vi "ubinary_load_control.vi"(8 "error in":errorcluster, 10 "file (use dialog)":path, 11 "VI":refnum<vi>) -> (0 "error out":errorcluster)   [LabVIEW 2012]
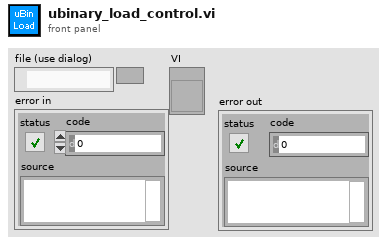
[diagram p1: front panel]
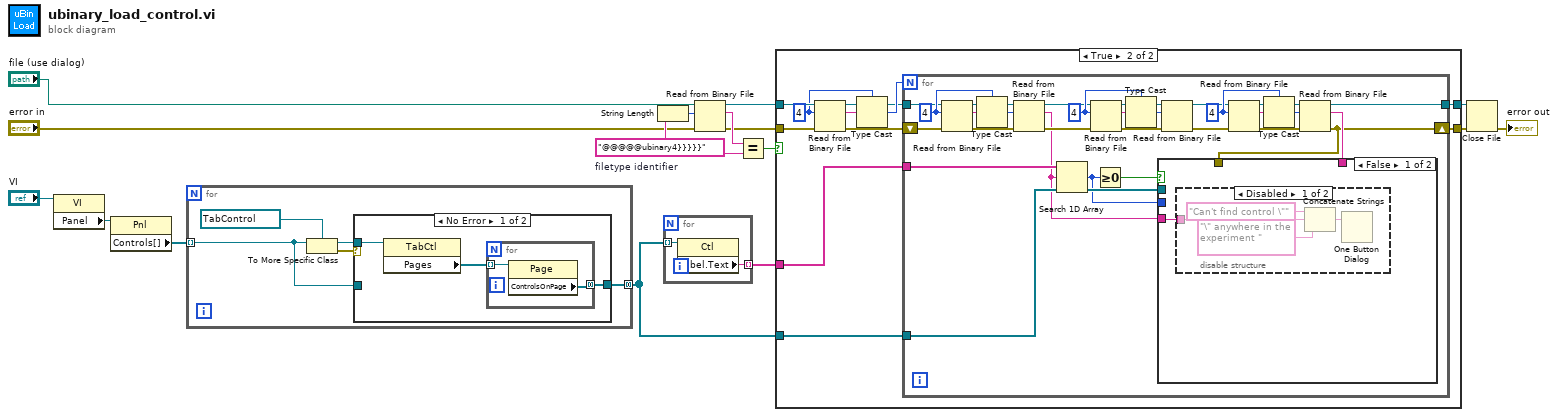
[diagram p0: block diagram]
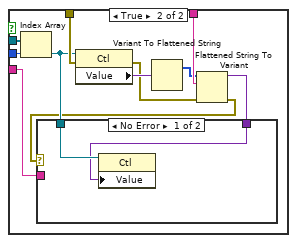
[diagram p4: hidden frame]
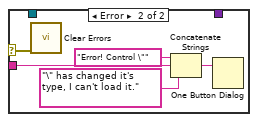
[diagram p5: hidden frame]
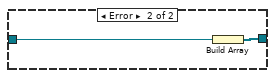
[diagram p6: hidden frame]
diagram:
  w11 = "@@@@@ubinary4}}}}}"  # filetype identifier
  n1 = property class="VI"(reference="VI") -> ("Panel"=w16:refnum<vi>)  [unwired: 1 in, 2 out]
  n2 = property class="Pnl"(reference=w16) -> ("Controls[]"=w15:refnum<vi>[])  [unwired: 1 in, 2 out]
  n3 = for {
    tunnel: w15 -> [w18] mode=indexing
    tunnel: [w17] -> w1 mode=concatenating
    n4 = To More Specific Class(target class=refnum<vi> refnum ("reference"), reference=w18) -> (specific class reference=w20:refnum<vi>, error out=w19:errorcluster)  [unwired: 1 in]
    n5 = case shown="No Error" w19 {
      tunnel: w20 -> [w24 _]
      tunnel: [w22 w28] -> w17
      tunnel: w18 -> [_ w27]
      frame No Error {
        n6 = property on="Property Node" class="TabCtl"(reference=w24) -> ("Pages"=w23:refnum<vi>[])  [unwired: 1 in, 2 out]
        n7 = for {
          tunnel: w23 -> [w26] mode=indexing
          tunnel: [w25] -> w22 mode=concatenating
          n8 = property class="Page"(reference=w26) -> ("ControlsOnPage"=w25:refnum<vi>[])  [unwired: 1 in, 2 out]
        }
      }
      frame Error {
        n9 = Build Array(w27) -> (w28:refnum<vi>[])
      }
    }
  }
  n10 = String Length(string=w11) -> (length=w12:i32)
  n11 = for {
    tunnel: w1 -> [w30] mode=indexing
    tunnel: [w29] -> w6 mode=indexing
    n12 = property class="Ctl"(reference=w30) -> ("Label.Text"=w29:string)  [unwired: 1 in, 2 out]
  }
  n13 = Read from Binary File(8:"error in", 10:w12, 11:"file (use dialog)") -> (0:w7:errorcluster, 2:w10:string, 3:w9:refnum<file>)  [unwired: 3 in, 1 out]
  n14 = Equal?(x=w10, y=w11) -> (x = y?=w8:bool)
  n15 = case shown="True" w8 {
    tunnel: [w32 w33] -> w13
    tunnel: w9 -> [w32 w43]
    tunnel: w7 -> [w31 w38]
    tunnel: w6 -> [_ w37]
    tunnel: [w31 w36] -> w5
    tunnel: w1 -> [_ w35]
    frame False {
    }
    frame True {
      w41 = 4 ("count (1)")
      n16 = Read from Binary File(8:w38, 10:w41, 11:w43) -> (0:w39:errorcluster, 2:w42:string, 3:w34:refnum<file>)  [unwired: 3 in, 1 out]
      n17 = Type Cast(type=w41, x=w42) -> (*(type *) &x=w40:i32)
      n18 = for {
        N: w40 -> [_]
        tunnel: w34 -> [w70]
        shift-right: [w44] -> w36
        shift-left: w39 -> [w66]
        tunnel: w37 -> [w65]
        tunnel: w35 -> [w49]
        tunnel: [w45] -> w33
        w59 = 4 ("count (1)")
        w60 = 4 ("count (1)")
        w72 = 4 ("count (1)")
        n19 = Read from Binary File(8:w66, 10:w72, 11:w70) -> (0:w67:errorcluster, 2:w71:string, 3:w69:refnum<file>)  [unwired: 3 in, 1 out]
        n20 = Type Cast(type=w72, x=w71) -> (*(type *) &x=w68:i32)
        n21 = Read from Binary File(8:w67, 10:w68, 11:w69) -> (0:w53:errorcluster, 2:w46:string, 3:w54:refnum<file>)  [unwired: 3 in, 1 out]
        n22 = Search 1D Array(1D array=w65, element=w46) -> (index of element=w48:i32)  [unwired: 1 in]
        n23 = Read from Binary File(8:w53, 10:w60, 11:w54) -> (0:w64:errorcluster, 2:w61:string, 3:w62:refnum<file>)  [unwired: 3 in, 1 out]
        n24 = Greater Or Equal To 0?(x=w48) -> (x >= 0?=w50:bool)
        n25 = Type Cast(type=w60, x=w61) -> (*(type *) &x=w63:i32)
        n26 = Read from Binary File(8:w64, 10:w63, 11:w62) -> (0:w52:errorcluster, 3:w51:refnum<file>)  [unwired: 3 in, 2 out]
        n27 = Read from Binary File(8:w52, 10:w59, 11:w51) -> (0:w55:errorcluster, 2:w58:string, 3:w57:refnum<file>)  [unwired: 3 in, 1 out]
        n28 = Type Cast(type=w59, x=w58) -> (*(type *) &x=w56:i32)
        n29 = Read from Binary File(8:w55, 10:w56, 11:w57) -> (0:w44:errorcluster, 2:w47:string, 3:w45:refnum<file>)  [unwired: 3 in, 1 out]
        n30 = case shown="False" w50 {
          tunnel: w49 -> [_ w88]
          tunnel: w48 -> [_ w87]
          tunnel: w47 -> [_ w86]
          tunnel: w46 -> [w73 w78]
          tunnel: w44 -> [_ w82]
          frame False {
            n31 = disable-structure shown="Disabled" {
              disable-tunnel: w73 -> [w77 _]
              frame Disabled {
                n32 = Concatenate Strings("Can't find control \"" ("string"), w77, "\" anywhere in the experiment " ("string")) -> (w76:string)
                n33 = One Button Dialog(message=w76) -> ()  [unwired: 1 in, 1 out]
              }
              frame Enabled {
              }
            }
          }
          frame True {
            n34 = Index Array(array=w88, index=w87) -> (element=w81:refnum<vi>)
            n35 = property class="Ctl"(reference=w81, error in=w82) -> (error out=w83:errorcluster, "Value"=w85:variant)  [unwired: 1 out]
            n36 = Variant To Flattened String(Variant=w85) -> (1:w84:i16[])  [unwired: 1 out]
            n37 = Flattened String To Variant(4:w83, 6:w86, 7:w84) -> (0:w80:errorcluster, 3:w79:variant)
            n38 = case shown="No Error" w80 {
              selector: w80 -> [_ w95]
              tunnel: w81 -> [w90 _]
              tunnel: w79 -> [w89 _]
              tunnel: w78 -> [_ w93]
              frame No Error {
                n39 = property class="Ctl"(reference=w90, "Value"=w89) -> ()  [unwired: 1 in, 2 out]
              }
              frame Error {
                n40 = call <vilib>:"Clear Errors.vi"("error in (no error)"=w95) -> ()  [unwired: 6 in, 1 out]
                n41 = Concatenate Strings("Error! Control \"" ("string"), w93, "\" has changed it's type, I can't load it." ("string")) -> (w94:string)
                n42 = One Button Dialog(message=w94) -> ()  [unwired: 1 in, 1 out]
              }
            }
          }
        }
      }
    }
  }
  n43 = Close File(refnum=w13, error in=w5) -> (error out=→"error out":errorcluster)  [unwired: 1 out]
